vi "GL_HeaterOn.vi"() -> ()   [LabVIEW 2019]
panel:
  out "HEATER ON":bool
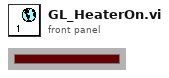
[diagram p1: front panel]
diagram:
